vi "Parse.vi"(8 "error in":errorcluster, 10 "Object Section":refnum<class "Section.lvclass">, 11 "Supported Objects in":refnum<class "Supported Objects.lvclass">) -> (0 "error out":errorcluster, 3 "Supported Objects out":refnum<class "Supported Objects.lvclass">)   [LabVIEW 2024, in "Electronic Datasheet.lvlib" / "Supported Objects.lvclass"]
uses:
  Supported Objects.lvclass
  OD Section/Section.lvclass
  OD Section/Section.lvclass/Section.ctl
  Supported Objects.lvclass/Supported Objects.ctl
  Keyname/Key Name.lvclass
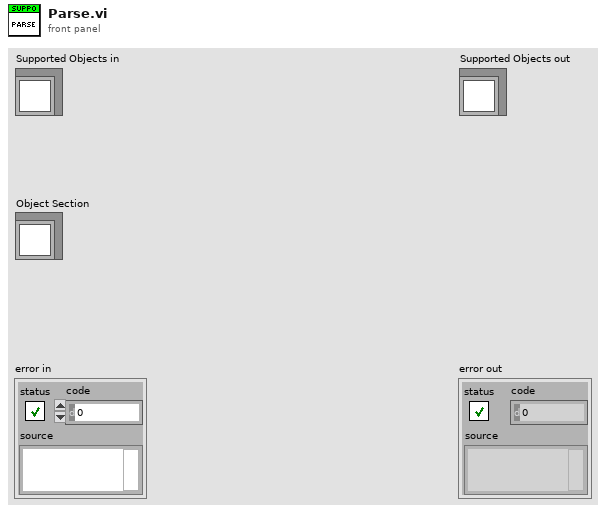
[diagram p1: front panel]
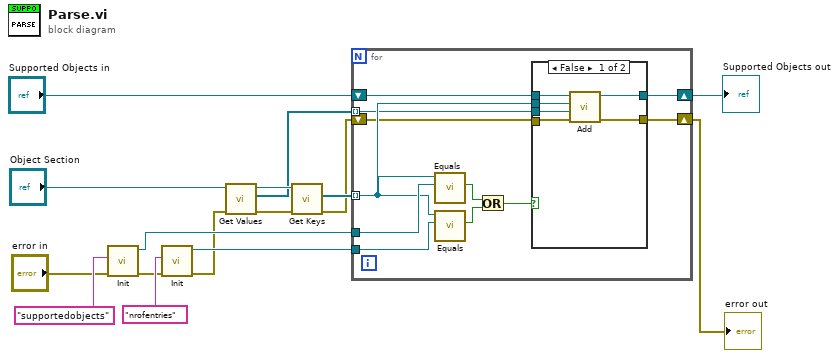
[diagram p0: block diagram]
diagram:
  n1 = call "Init.vi"("error in"="error in", "Key Name"="supportedobjects") -> ("error out"=w7:errorcluster, "Key Name out"=w12:refnum<class "Key Name.lvclass">)  [unwired: 8 in]
  n2 = call "Init.vi"("error in"=w7, "Key Name"="nrofentries") -> ("error out"=w6:errorcluster, "Key Name out"=w10:refnum<class "Key Name.lvclass">)  [unwired: 8 in]
  n3 = call "Get Values.vi"("error in (no error)"=w6, "Section in"="Object Section") -> ("error out"=w5:errorcluster, "Values"=w2:refnum<class "Value.lvclass">[], "Section out"=w3:refnum<class "Section.lvclass">)  [unwired: 7 in]
  n4 = call "Get Keys.vi"("error in"=w5, "Object Entry in"=w3) -> ("error out"=w1:errorcluster, "Keys"=w16:refnum<class "Key Name.lvclass">[])  [unwired: 7 in, 1 out]
  n5 = for {
    tunnel: w16 -> [w22] mode=indexing
    shift-right: [w26] -> w14
    shift-left: "Supported Objects in" -> [w27]
    tunnel: w12 -> [w23]
    tunnel: w10 -> [w21]
    shift-right: [w19] -> w9
    shift-left: w1 -> [w18]
    tunnel: w2 -> [w17] mode=indexing
    n6 = call "Equals.vi"("Keyname"=w23, "Keyname in"=w22) -> ("Equal?"=w24:bool)  [unwired: 8 in, 1 out]
    n7 = call "Equals.vi"("Keyname"=w21, "Keyname in"=w22) -> ("Equal?"=w20:bool)  [unwired: 8 in, 1 out]
    n8 = Or(x=w24, y=w20) -> (x .or. y?=w25:bool)
    n9 = case shown="False" w25 {
      tunnel: w27 -> [w33 w35]
      tunnel: [w32 w35] -> w26
      tunnel: w22 -> [w31 _]
      tunnel: [w30 w34] -> w19
      tunnel: w18 -> [w29 w34]
      tunnel: w17 -> [w28 _]
      frame False {
        n10 = call "Add.vi"("error in"=w29, "Value"=w28, "Key"=w31, "Supported Objects in"=w33) -> ("error out"=w30:errorcluster, "Supported Objects out"=w32:refnum<class "Supported Objects.lvclass">)  [unwired: 6 in]
      }
      frame True {
      }
    }
  }
  "error out" <- w9
  "Supported Objects out" <- w14
